vi "Auto Choose Resource.vi"(8 "error in (no error)":errorcluster, 11 "RP2040.lvlib:RP2040Platform in":refnum<class "RP2040Platform.lvclass">) -> (0 "error out":errorcluster, 1 "Cancelled":bool, 2 "Resource":refnum<class "DeployResource.lvclass">, 3 "RP2040.lvlib:RP2040Platform out":refnum<class "RP2040Platform.lvclass">)   [LabVIEW 2020, in "RP2040.lvlib" / "RP2040Platform.lvclass"]
uses:
  RP2040Platform.lvclass
  Builds/picoG/ppl/PicoG-Core.lvlibp/DeployResource/DeployResource.lvclass
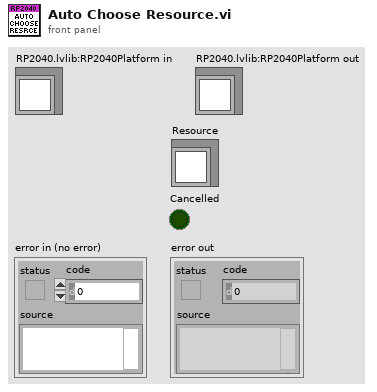
[diagram p1: front panel]
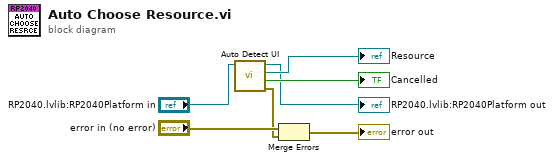
[diagram p0: block diagram]
diagram:
  n1 = call "Auto Detect UI.vi"("RP2040.lvlib:RP2040Platform in"="RP2040.lvlib:RP2040Platform in") -> ("error out"=w3:errorcluster, "Cancelled"=→"Cancelled":bool, "Resource"=→"Resource":refnum<class "DeployResource.lvclass">, "RP2040.lvlib:RP2040Platform out"=→"RP2040.lvlib:RP2040Platform out":refnum<class "RP2040Platform.lvclass">)  [unwired: 7 in]
  n2 = Merge Errors("error in (no error)", w3) -> (→"error out":errorcluster)
